vi "get_reference_fns.vi"(9 "Central wavelength (nm)":dbl, 10 "Gamma":dbl, 11 "Alpha":dbl) -> (1 "reference":string, 2 "second derivative reference":T1, 3 "reference":T1, 4 "second derivative reference":string)   [LabVIEW 2022 SP3]
uses:
  <vilib>/gmath/NI_Gmath.lvlib
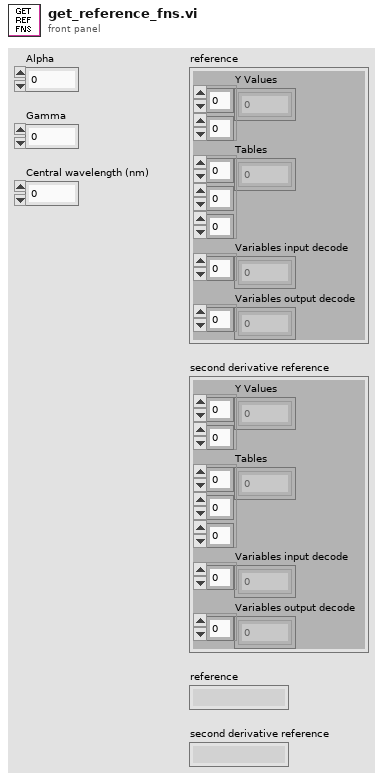
[diagram p1: front panel]
types:
  T1 = cluster{"Y Values":dbl[][], "Tables":i32[][][], "Variables input decode":i32[], "Variables output decode":i32[]}
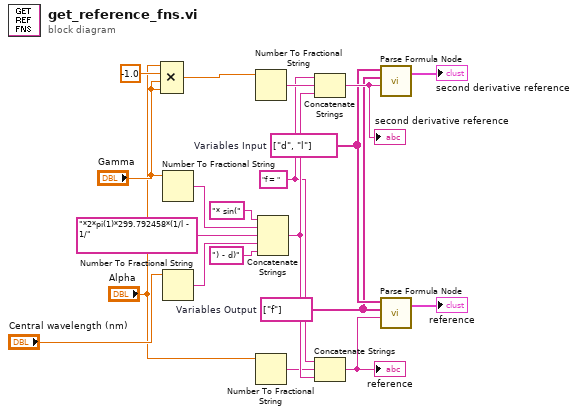
[diagram p0: block diagram]
diagram:
  w10 = "f = " ("string")
  w3 = string[] ["f"]  # Variables Output
  w4 = string[] ["d", "l"]  # Variables Input
  n1 = Compound Arithmetic op=MULTIPLY("Alpha", -1.0, "Gamma", "Gamma") -> (w16:dbl)
  n2 = Number To Fractional String(number="Gamma") -> (F-format string=w8:string)  [unwired: 3 in]
  n3 = Number To Fractional String(number="Central wavelength (nm)") -> (F-format string=w18:string)  [unwired: 3 in]
  n4 = Number To Fractional String(number=w16) -> (F-format string=w15:string)  [unwired: 3 in]
  n5 = Number To Fractional String(number="Alpha") -> (F-format string=w5:string)  [unwired: 3 in]
  n6 = Concatenate Strings("* sin(" ("string"), w8, "*2*pi(1)*299.792458*(1/l - 1/" ("string"), w18, ") - d)" ("string")) -> (w11:string)
  n7 = Concatenate Strings(w10, w15, w11) -> (w12:string)
  "second derivative reference" <- w12
  n8 = Concatenate Strings(w10, w5, w11) -> (w6:string)
  "reference" <- w6
  n9 = call <vilib>:"Parse Formula Node.vi"("formula"=w12, "Variables Output"=w3, "Variables Input"=w4) -> ("Parsed Formula Node"=→"second derivative reference":T1)  [unwired: 1 in, 1 out]
  n10 = call <vilib>:"Parse Formula Node.vi"("formula"=w6, "Variables Output"=w3, "Variables Input"=w4) -> ("Parsed Formula Node"=→"reference":T1)  [unwired: 1 in, 1 out]
